vi "Main.vi"() -> ()   [LabVIEW 2017]
uses:
  1. CTL/State.ctl
  <vilib>/Utility/sysdir.llb/System Directory Type.ctl
  <vilib>/Instr/_visa.llb/VISA Configure Serial Port (Instr).vi
panel:
  in  "VISA resource name":refnum<visa-resource-name> caption="VISA 리소스 이름"
  out "String 3":string
  out "String 2":string
  out "String":string
  out "3회시험결과":string
  out "2회시험결과":string
  out "1회시험결과":string
  out "시험결과":string
  in  "데이터 저장":bool=TRUE
  in  "PNF ON":bool=TRUE
  in  "정지 버튼":bool=TRUE
  # "AUV Pinger TEST"
  # "시험 결과"
  # "COM 포트 설정"
  # "1회 시험 데이터"
  # "2회 시험 데이터"
  # "3회 시험 데이터"
  # "2회 시험 결과"
  # "3회 시험 결과"
  # "1회 시험 결과"
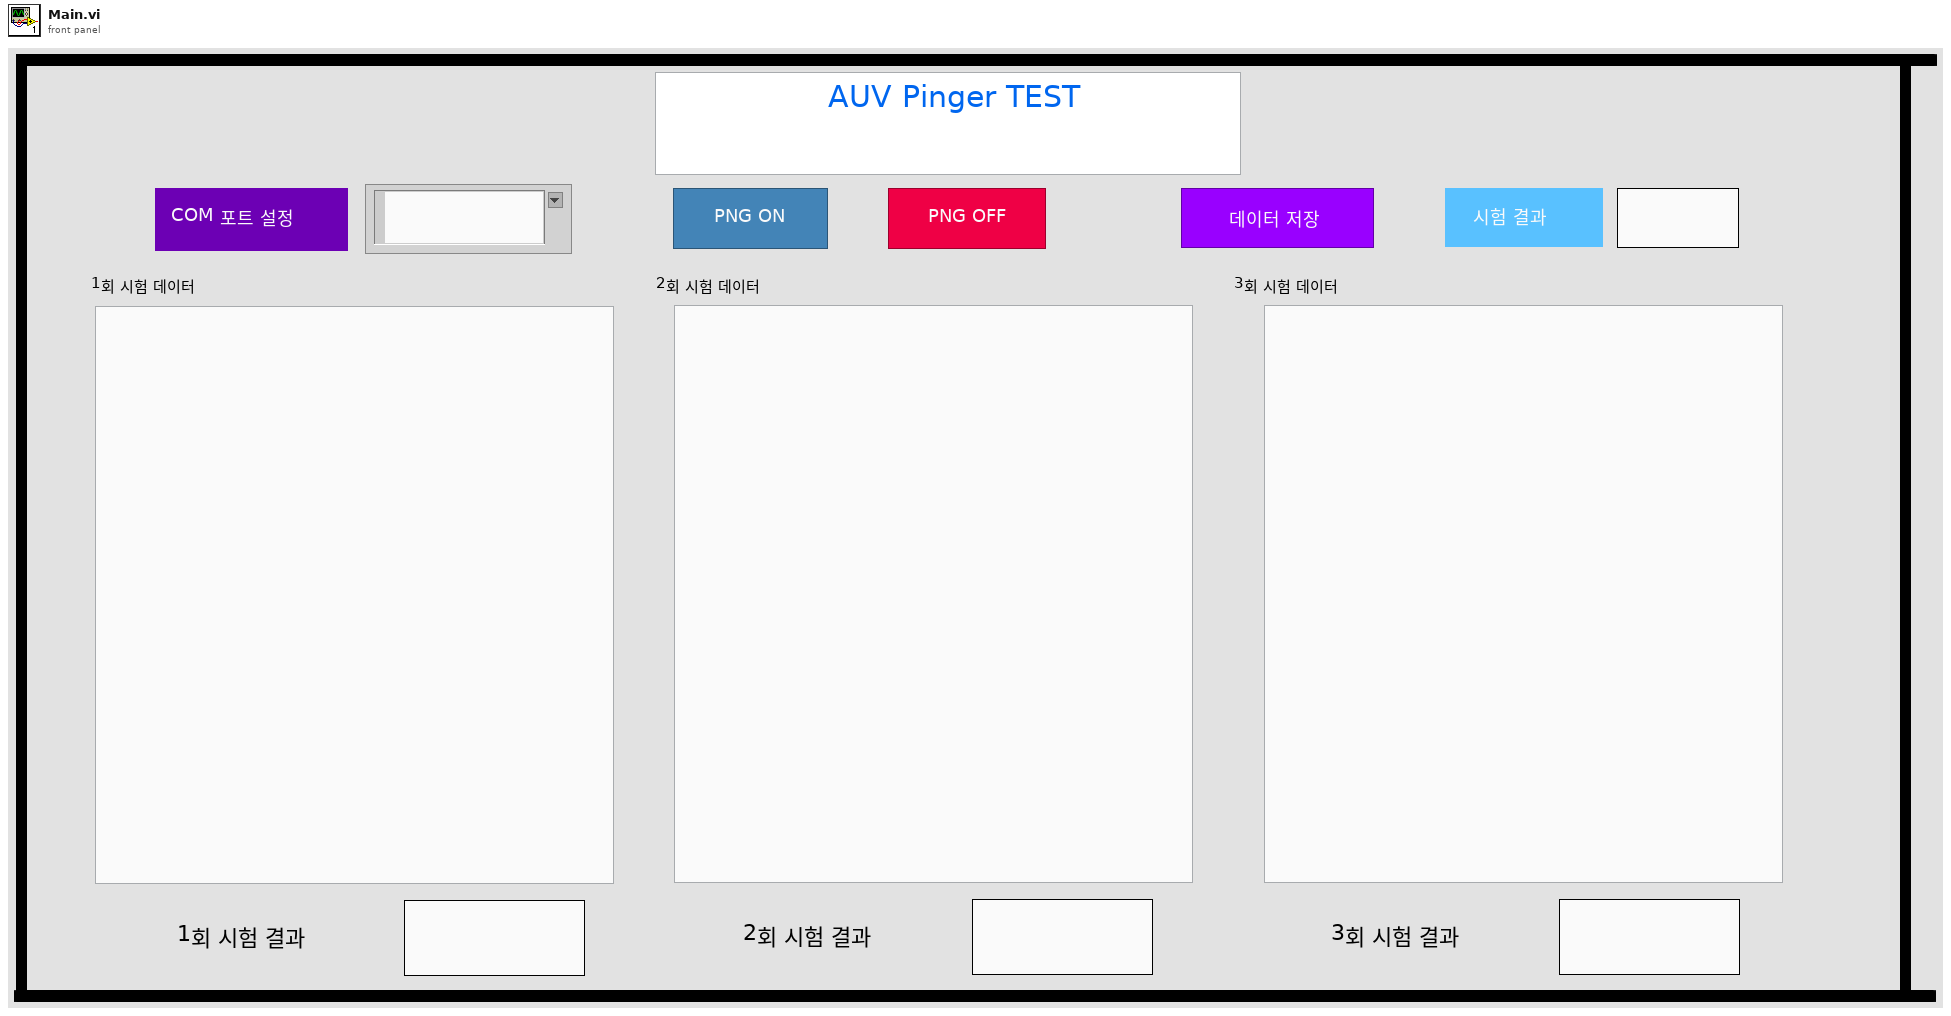
[diagram p1: front panel]
types:
  T1 = cluster{"1회 시험결과":string, "2회 시험결과":string, "3회 시험결과":string, "시험결과":string, "COM 포트":refnum<visa-resource-name>, "카운터":i32, "1회 로그":string, "2회 로그":string, "3회 로그":string, "1회 결과 카운트":i32, "2회 결과 카운트":i32, "3회 결과 카운트":i32}
  T2 = typedef "State.ctl" = enum16{"초기화", "시작", "정지", "데이터 저장"}
  T3 = enum16{"open", "replace", "create", "open or create", "replace or create", "replace or create with confirmation"}
  T4 = typedef "System Directory Type.ctl" = i32
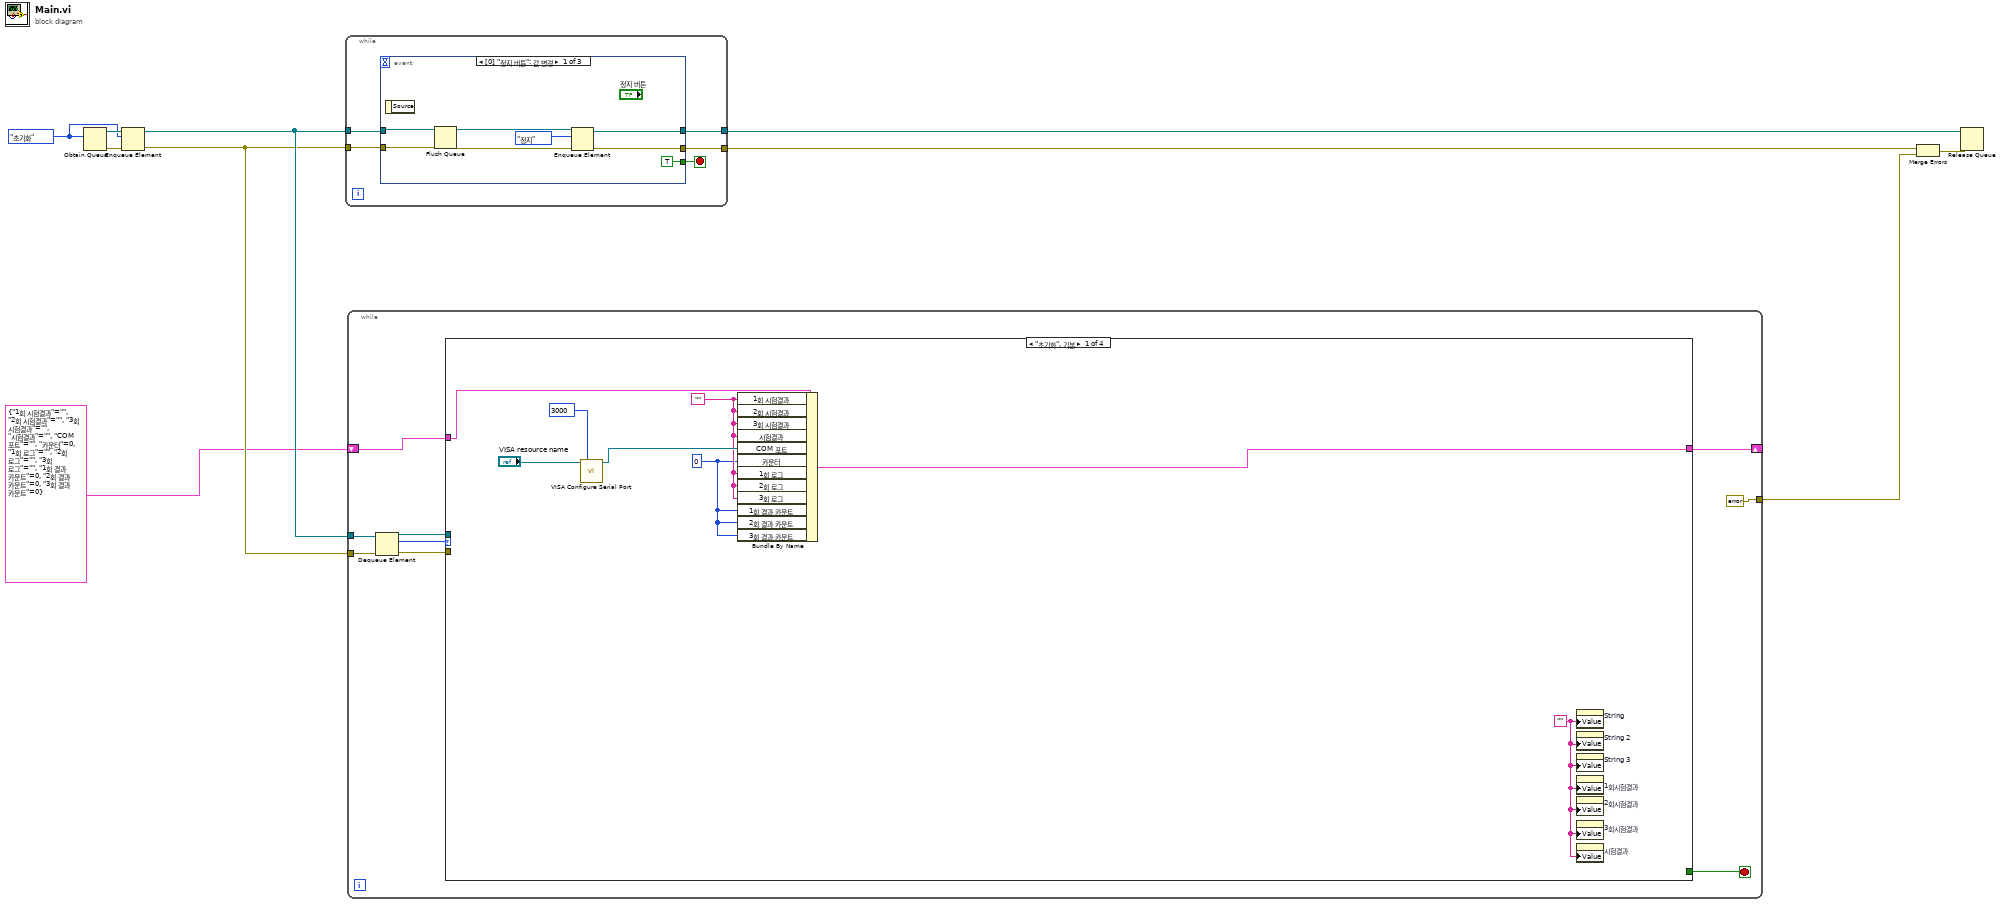
[diagram p0: block diagram]
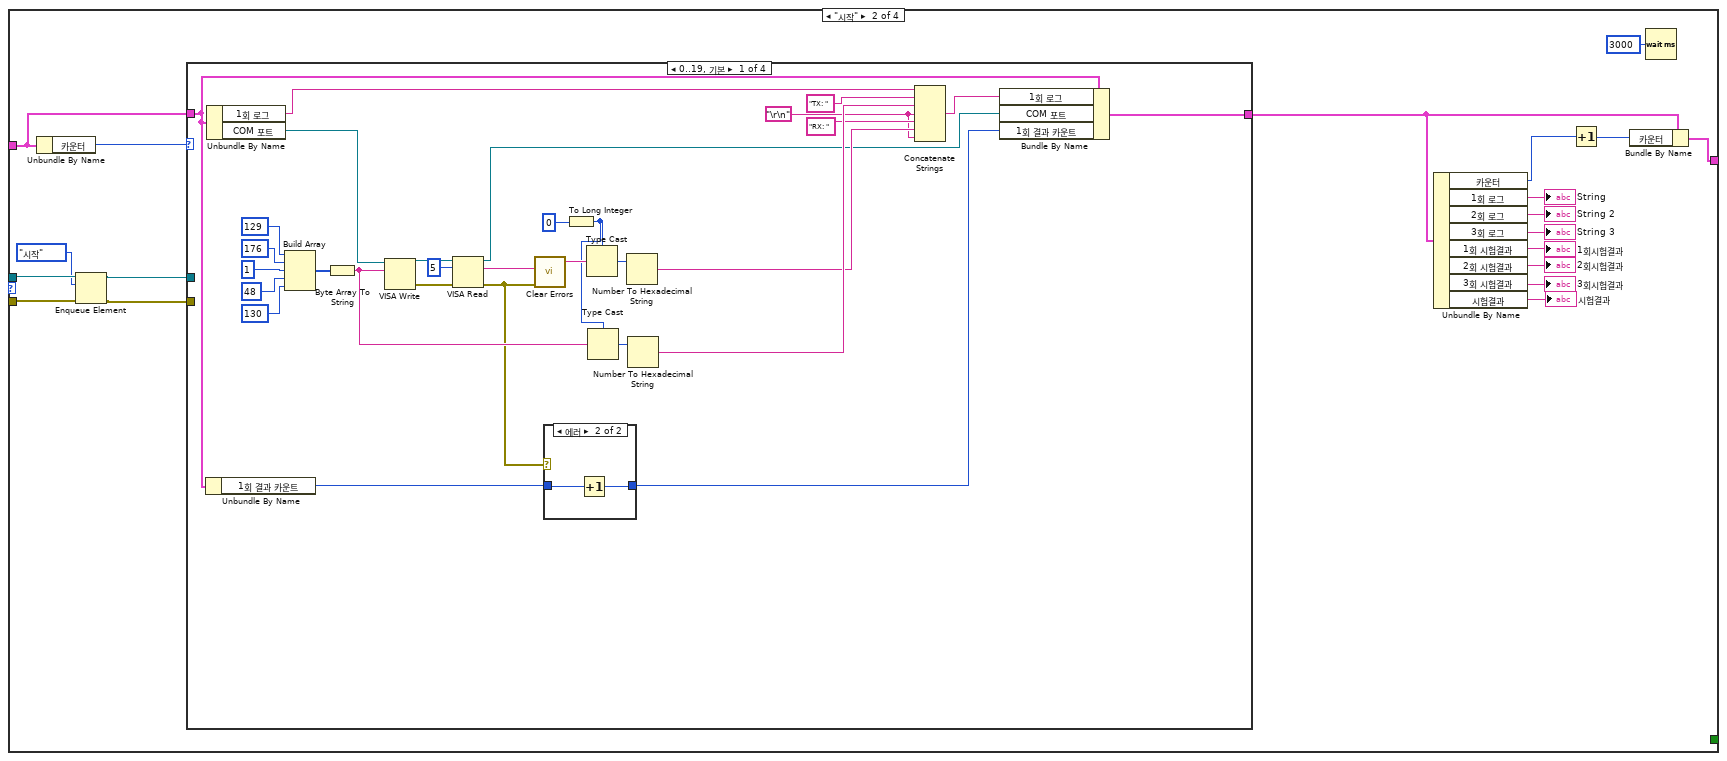
[diagram p2: hidden frame]
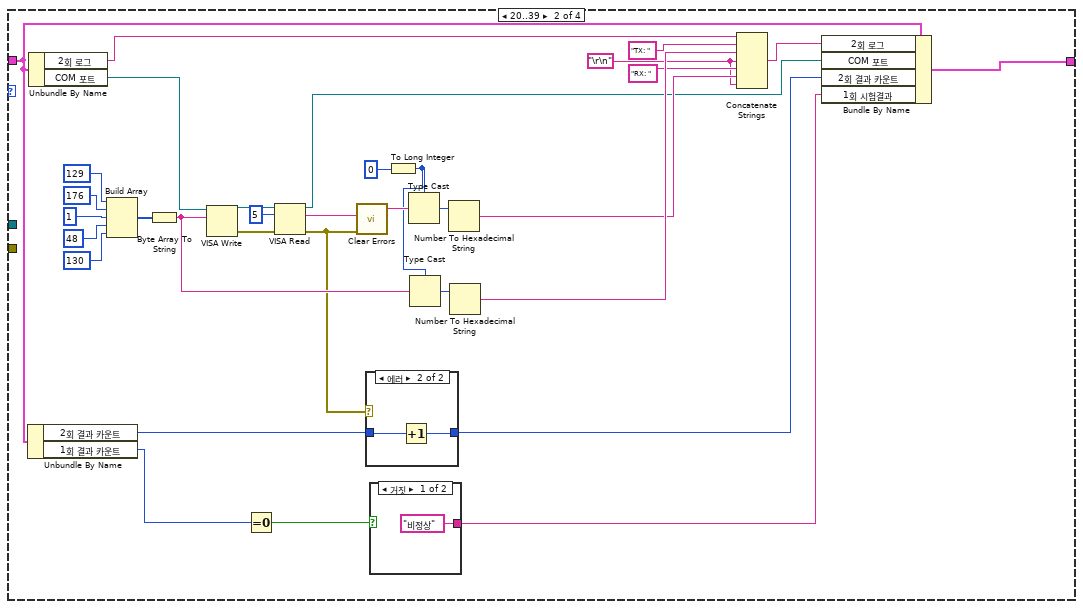
[diagram p4: hidden frame]
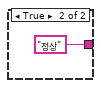
[diagram p5: hidden frame]
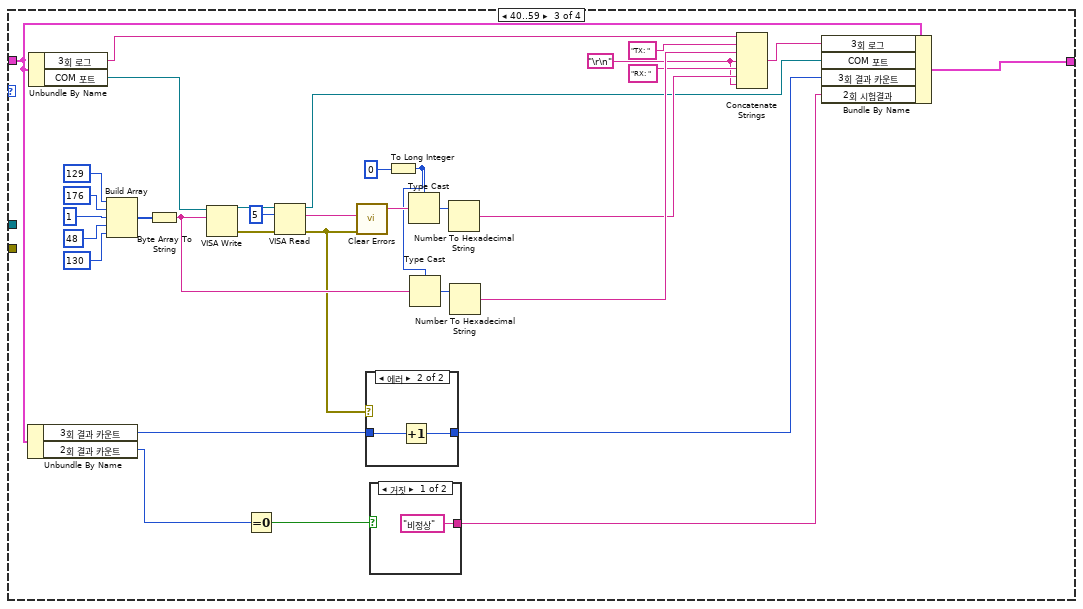
[diagram p7: hidden frame]
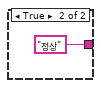
[diagram p8: hidden frame]
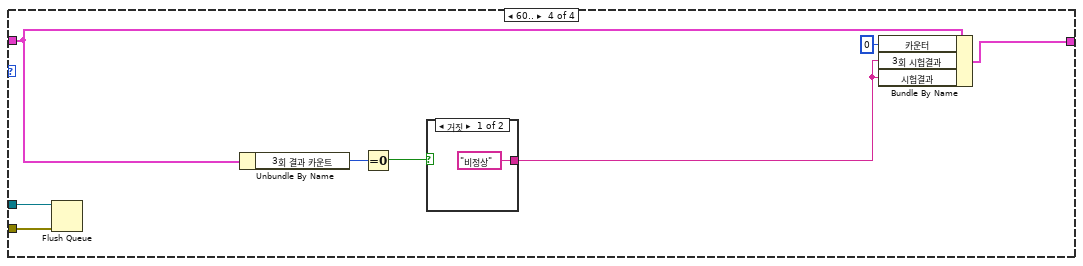
[diagram p10: hidden frame]
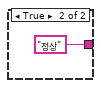
[diagram p11: hidden frame]
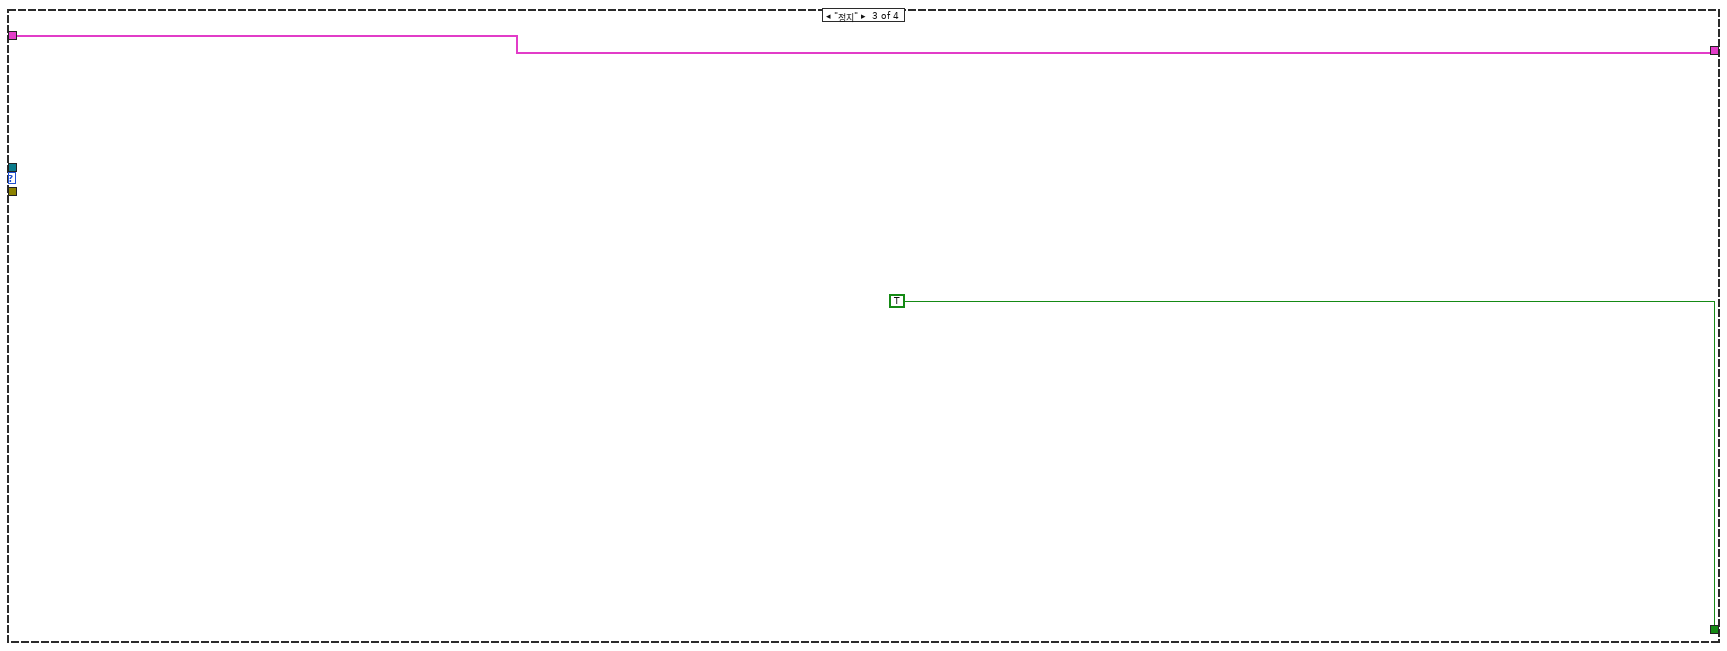
[diagram p12: hidden frame]
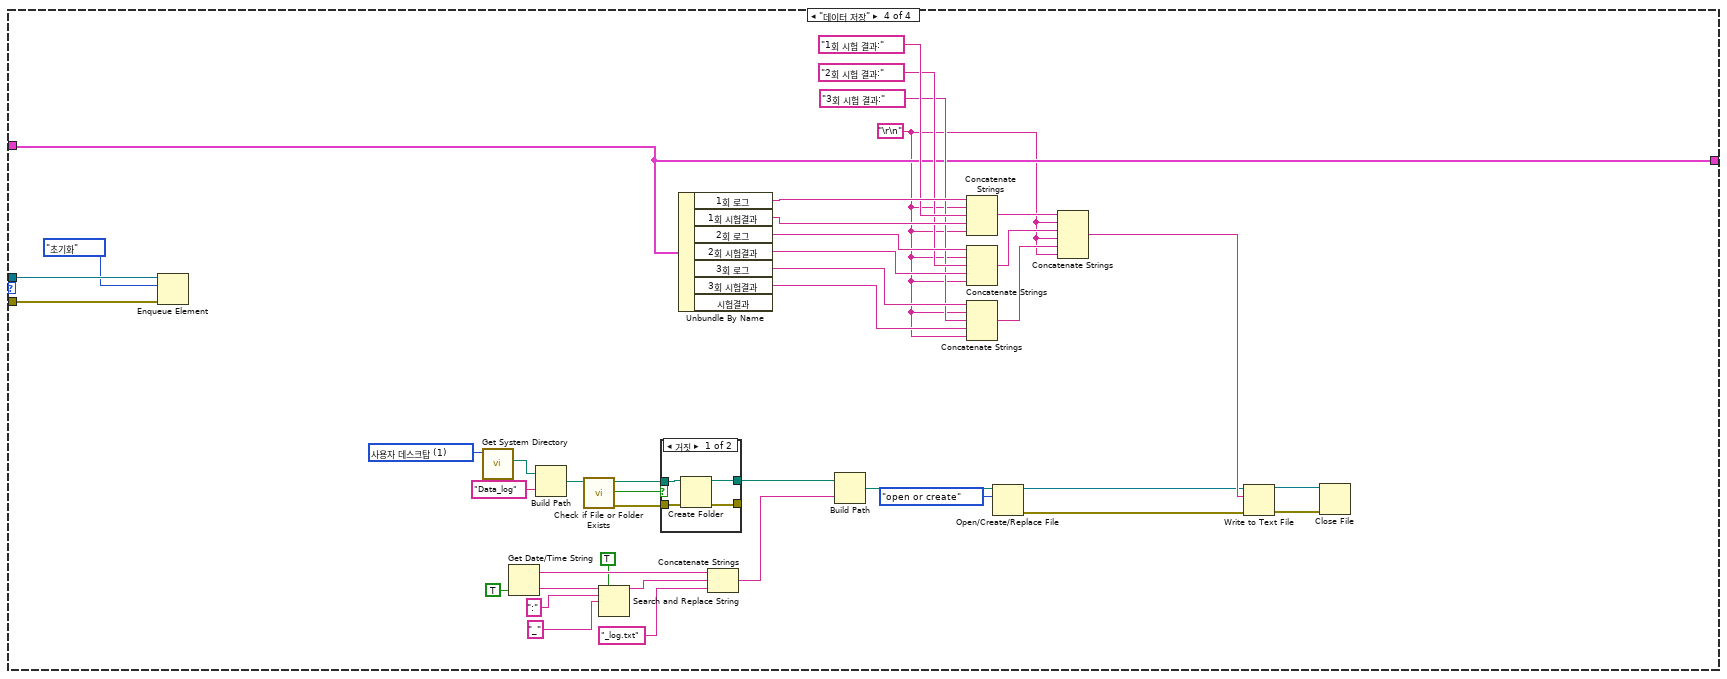
[diagram p13: hidden frame]
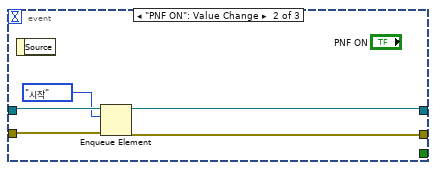
[diagram p15: hidden frame]
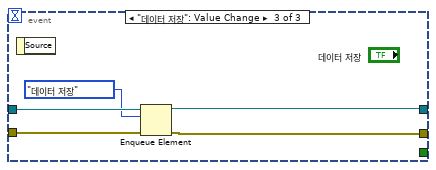
[diagram p16: hidden frame]
diagram:
  w8 = State."초기화"
  n1 = Obtain Queue(element data type=w8) -> (queue out=w10:refnum<queue>, error out=w9:errorcluster)  [unwired: 4 in, 1 out]
  n2 = Enqueue Element(queue=w10, element=w8, error in (no error)=w9) -> (queue out=w7:refnum<queue>, error out=w6:errorcluster)  [unwired: 1 in, 1 out]
  n3 = while {
    tunnel: w7 -> [w15]
    tunnel: w6 -> [w14]
    tunnel: [w12] -> w5
    tunnel: [w11] -> w2
    stop <- w13 stop-if-true
    n4 = event shown="[0] \"정지 버튼\": 값 변경" {
      selector: _ -> [_ _ _]
      dyn-events: _ -> [_ _ _]
      timeout: _ -> [_ _ _]
      tunnel: w15 -> [w16 w28 w33]
      tunnel: w14 -> [w17 w27 w32]
      tunnel: [TRUE _ _] -> w13
      tunnel: [w21 w24 w29] -> w12
      tunnel: [w20 w25 w30] -> w11
      event "정지 버튼": Value Change {
        n5 = event-data() -> ()  [unwired: 1 in, 1 out]
        n6 = Flush Queue(queue=w16, error in (no error)=w17) -> (queue out=w19:refnum<queue>, error out=w18:errorcluster)  [unwired: 1 out]
        n7 = Enqueue Element(queue=w19, element=State."정지", error in (no error)=w18) -> (queue out=w20:refnum<queue>, error out=w21:errorcluster)  [unwired: 1 in, 1 out]
      }
      event "PNF ON": Value Change {
        n8 = event-data() -> ()  [unwired: 1 in, 1 out]
        n9 = Enqueue Element(queue=w28, element=State."시작", error in (no error)=w27) -> (queue out=w25:refnum<queue>, error out=w24:errorcluster)  [unwired: 1 in, 1 out]
      }
      event "데이터 저장": Value Change {
        n10 = event-data() -> ()  [unwired: 1 in, 1 out]
        n11 = Enqueue Element(queue=w33, element=State."데이터 저장", error in (no error)=w32) -> (queue out=w30:refnum<queue>, error out=w29:errorcluster)  [unwired: 1 in, 1 out]
      }
    }
  }
  n12 = while {
    tunnel: w7 -> [w38]
    tunnel: w6 -> [w42]
    tunnel: [errorcluster {"status"=FALSE, "code"=0, "source"=""} ("에러 상수")] -> w4
    shift-right: [w34] -> _
    shift-left: T1 {"1회 시험결과"="", "2회 시험결과"="", "3회 시험결과"="", "시험결과"="", "COM 포트"="", "카운터"=0, "1회 로그"="", "2회 로그"="", "3회 로그"="", "1회 결과 카운트"=0, "2회 결과 카운트"=0, "3회 결과 카운트"=0} -> [w39]
    stop <- w41 stop-if-true
    n13 = Dequeue Element(queue=w38, error in (no error)=w42) -> (queue out=w36:refnum<queue>, element=w37:T2, error out=w35:errorcluster)  [unwired: 1 in, 1 out]
    n14 = case shown="\"초기화\", 기본" w37 {
      tunnel: [_ _ TRUE _] -> w41
      tunnel: w39 -> [w50 w68 w186 w204]
      tunnel: [w49 w61 w186 w204] -> w34
      tunnel: w36 -> [_ w60 _ w228]
      tunnel: w35 -> [_ w59 _ w227]
      frame "초기화", Default {
        w43 = 0
        w44 = ""
        w45 = ""
        n15 = call-poly "VISA Configure Serial Port"("VISA resource name"="VISA resource name", "timeout (10sec)"=u32 3000) -> ("VISA resource name out"=w47:refnum<visa-resource-name>)  [unwired: 12 in, 1 out]
        n16 = Bundle By Name(cluster=w50, "1회 시험결과"=w44, "2회 시험결과"=w44, "3회 시험결과"=w44, "시험결과"=w44, "COM 포트"=w47, "카운터"=w43, "1회 로그"=w44, "2회 로그"=w44, "3회 로그"=w44, "1회 결과 카운트"=w43, "2회 결과 카운트"=w43, "3회 결과 카운트"=w43) -> (w49:T1)
        n17 = property on="String" class="Str"("Value"=w45) -> ()  [unwired: 2 in, 2 out]
        n18 = property on="String 2" class="Str"("Value"=w45) -> ()  [unwired: 2 in, 2 out]
        n19 = property on="String 3" class="Str"("Value"=w45) -> ()  [unwired: 2 in, 2 out]
        n20 = property on="1회시험결과" class="Str"("Value"=w45) -> ()  [unwired: 2 in, 2 out]
        n21 = property on="2회시험결과" class="Str"("Value"=w45) -> ()  [unwired: 2 in, 2 out]
        n22 = property on="3회시험결과" class="Str"("Value"=w45) -> ()  [unwired: 2 in, 2 out]
        n23 = property on="시험결과" class="Str"("Value"=w45) -> ()  [unwired: 2 in, 2 out]
      }
      frame "시작" {
        n24 = Unbundle By Name(w68) -> ("카운터"=w69:i32)
        n25 = Enqueue Element(queue=w60, element=State."시작", error in (no error)=w59) -> (queue out=w57:refnum<queue>, error out=w56:errorcluster)  [unwired: 1 in, 1 out]
        n26 = case shown="0..19, 기본" w69 {
          tunnel: w68 -> [w72 w107 w144 w181]
          tunnel: [w97 w132 w169 w182] -> w66
          tunnel: w57 -> [_ _ _ w177]
          tunnel: w56 -> [_ _ _ w176]
          frame 0..19, Default {
            w77 = "\r\n"
            n27 = Unbundle By Name(w72) -> ("1회 결과 카운트"=w71:i32)
            n28 = Unbundle By Name(w72) -> ("1회 로그"=w84:string, "COM 포트"=w83:refnum<visa-resource-name>)
            n29 = Build Array(129, 176, 1, 48, 130) -> (w88:i32[])
            n30 = Byte Array To String(unsigned byte array=w88) -> (string=w82:string)
            n31 = VISA Write(VISA resource name=w83, write buffer=w82) -> (VISA resource name out=w96:refnum<visa-resource-name>, error out=w94:errorcluster)  [unwired: 1 in, 1 out]
            n32 = VISA Read(VISA resource name=w96, byte count=u32 5 ("바이트 카운트"), error in (no error)=w94) -> (VISA resource name out=w76:refnum<visa-resource-name>, read buffer=w87:string, error out=w73:errorcluster)  [unwired: 1 out]
            n33 = call <vilib>:"Clear Errors.vi"("error in (no error)"=w73) -> ()  [unwired: 5 in, 2 out]
            n34 = case shown="에러" w73 {
              tunnel: [w99 w101] -> w70
              tunnel: w71 -> [w99 w100]
              frame No Error {
              }
              frame Error {
                n35 = Increment(x=w100) -> (x+1=w101:i32)
              }
            }
            n36 = To Long Integer(number=0 ("숫자")) -> (32bit integer=w75:i32)
            n37 = Type Cast(type=w75, x=w87) -> (*(type *) &x=w86:i32)
            n38 = Type Cast(type=w75, x=w82) -> (*(type *) &x=w74:i32)
            n39 = Number To Hexadecimal String(2:w86) -> (0:w78:string)  [unwired: 1 in]
            n40 = Number To Hexadecimal String(2:w74) -> (0:w80:string)  [unwired: 1 in]
            n41 = Concatenate Strings(w84, "TX: ", w80, w77, "RX: ", w78, w77) -> (w98:string)
            n42 = Bundle By Name(cluster=w72, "1회 로그"=w98, "COM 포트"=w76, "1회 결과 카운트"=w70) -> (w97:T1)
          }
          frame 20..39 {
            w112 = "\r\n"
            n43 = Unbundle By Name(w107) -> ("2회 결과 카운트"=w106:i32, "1회 결과 카운트"=w104:i32)
            n44 = Unbundle By Name(w107) -> ("2회 로그"=w119:string, "COM 포트"=w118:refnum<visa-resource-name>)
            n45 = Build Array(129, 176, 1, 48, 130) -> (w123:i32[])
            n46 = Byte Array To String(unsigned byte array=w123) -> (string=w117:string)
            n47 = VISA Write(VISA resource name=w118, write buffer=w117) -> (VISA resource name out=w131:refnum<visa-resource-name>, error out=w129:errorcluster)  [unwired: 1 in, 1 out]
            n48 = Equal To 0?(x=w104) -> (x = 0?=w103:bool)
            n49 = VISA Read(VISA resource name=w131, byte count=u32 5 ("바이트 카운트"), error in (no error)=w129) -> (VISA resource name out=w111:refnum<visa-resource-name>, read buffer=w122:string, error out=w108:errorcluster)  [unwired: 1 out]
            n50 = call <vilib>:"Clear Errors.vi"("error in (no error)"=w108) -> ()  [unwired: 5 in, 2 out]
            n51 = case shown="에러" w108 {
              tunnel: [w136 w138] -> w105
              tunnel: w106 -> [w136 w137]
              frame No Error {
              }
              frame Error {
                n52 = Increment(x=w137) -> (x+1=w138:i32)
              }
            }
            n53 = case shown="거짓" w103 {
              tunnel: ["비정상" "정상"] -> w102
              frame False {
              }
              frame True {
              }
            }
            n54 = To Long Integer(number=0 ("숫자")) -> (32bit integer=w110:i32)
            n55 = Type Cast(type=w110, x=w122) -> (*(type *) &x=w121:i32)
            n56 = Type Cast(type=w110, x=w117) -> (*(type *) &x=w109:i32)
            n57 = Number To Hexadecimal String(2:w121) -> (0:w113:string)  [unwired: 1 in]
            n58 = Number To Hexadecimal String(2:w109) -> (0:w115:string)  [unwired: 1 in]
            n59 = Concatenate Strings(w119, "TX: ", w115, w112, "RX: ", w113, w112) -> (w133:string)
            n60 = Bundle By Name(cluster=w107, "2회 로그"=w133, "COM 포트"=w111, "2회 결과 카운트"=w105, "1회 시험결과"=w102) -> (w132:T1)
          }
          frame 40..59 {
            w149 = "\r\n"
            n61 = Unbundle By Name(w144) -> ("3회 결과 카운트"=w143:i32, "2회 결과 카운트"=w141:i32)
            n62 = Unbundle By Name(w144) -> ("3회 로그"=w156:string, "COM 포트"=w155:refnum<visa-resource-name>)
            n63 = Build Array(129, 176, 1, 48, 130) -> (w160:i32[])
            n64 = Byte Array To String(unsigned byte array=w160) -> (string=w154:string)
            n65 = VISA Write(VISA resource name=w155, write buffer=w154) -> (VISA resource name out=w168:refnum<visa-resource-name>, error out=w166:errorcluster)  [unwired: 1 in, 1 out]
            n66 = Equal To 0?(x=w141) -> (x = 0?=w140:bool)
            n67 = VISA Read(VISA resource name=w168, byte count=u32 5 ("바이트 카운트"), error in (no error)=w166) -> (VISA resource name out=w148:refnum<visa-resource-name>, read buffer=w159:string, error out=w145:errorcluster)  [unwired: 1 out]
            n68 = call <vilib>:"Clear Errors.vi"("error in (no error)"=w145) -> ()  [unwired: 5 in, 2 out]
            n69 = case shown="에러" w145 {
              tunnel: [w173 w175] -> w142
              tunnel: w143 -> [w173 w174]
              frame No Error {
              }
              frame Error {
                n70 = Increment(x=w174) -> (x+1=w175:i32)
              }
            }
            n71 = case shown="거짓" w140 {
              tunnel: ["비정상" "정상"] -> w139
              frame False {
              }
              frame True {
              }
            }
            n72 = To Long Integer(number=0 ("숫자")) -> (32bit integer=w147:i32)
            n73 = Type Cast(type=w147, x=w159) -> (*(type *) &x=w158:i32)
            n74 = Type Cast(type=w147, x=w154) -> (*(type *) &x=w146:i32)
            n75 = Number To Hexadecimal String(2:w158) -> (0:w150:string)  [unwired: 1 in]
            n76 = Number To Hexadecimal String(2:w146) -> (0:w152:string)  [unwired: 1 in]
            n77 = Concatenate Strings(w156, "TX: ", w152, w149, "RX: ", w150, w149) -> (w170:string)
            n78 = Bundle By Name(cluster=w144, "3회 로그"=w170, "COM 포트"=w148, "3회 결과 카운트"=w142, "2회 시험결과"=w139) -> (w169:T1)
          }
          frame 60.. {
            n79 = Flush Queue(queue=w177, error in (no error)=w176) -> ()  [unwired: 3 out]
            n80 = Unbundle By Name(w181) -> ("3회 결과 카운트"=w180:i32)
            n81 = Equal To 0?(x=w180) -> (x = 0?=w179:bool)
            n82 = case shown="거짓" w179 {
              tunnel: ["비정상" "정상"] -> w178
              frame False {
              }
              frame True {
              }
            }
            n83 = Bundle By Name(cluster=w181, "카운터"=0, "3회 시험결과"=w178, "시험결과"=w178) -> (w182:T1)
          }
        }
        n84 = Unbundle By Name(w66) -> ("카운터"=w67:i32, "1회 로그"=→"String":string, "2회 로그"=→"String 2":string, "3회 로그"=→"String 3":string, "1회 시험결과"=→"1회시험결과":string, "2회 시험결과"=→"2회시험결과":string, "3회 시험결과"=→"3회시험결과":string, "시험결과"=→"시험결과":string)
        n85 = Increment(x=w67) -> (x+1=w65:i32)
        n86 = Bundle By Name(cluster=w66, "카운터"=w65) -> (w61:T1)
        n87 = Wait (ms)(milliseconds to wait=u32 3000 ("대기 시간 (ms)")) -> ()  [unwired: 1 out]
      }
      frame "정지" {
      }
      frame "데이터 저장" {
        w188 = "\r\n"
        w225 = T4 1 items=["사용자 홈"=0, "사용자 데스크탑"=1, "사용자 문서"=2, "사용자 어플리케이션 데이터"=3, "사용자 환경"=4, "사용자 임시"=5, "퍼블릭 문서"=6, "퍼블릭 어플리케이션 데이터"=7, "퍼블릭 환경"=8, "퍼블릭 캐시"=13, "시스템 코어 라이브러리"=9, "시스템 설치된 라이브러리"=10, "어플리케이션 파일"=11, "부팅 볼륨 루트"=12] ("system directory type")
        n88 = Enqueue Element(queue=w228, element=State."초기화", error in (no error)=w227) -> ()  [unwired: 1 in, 3 out]
        n89 = call <vilib>:"Get System Directory.vi"("system directory type"=w225) -> ("system directory"=w224:path)  [unwired: 10 in]
        n90 = Get Date/Time String(want seconds? (F)=TRUE ("초 보이기? (거짓)")) -> (date string=w193:string, time string=w197:string)  [unwired: 2 in]
        n91 = Build Path(base path=w224, name or relative path="Data_log" ("이름 또는 상대 경로")) -> (appended path=w222:path)
        n92 = call <vilib>:"Check if File or Folder Exists.vi"("path"=w222) -> ("error out"=w219:errorcluster, "file or folder exists?"=w221:bool, "dup path"=w220:path)  [unwired: 8 in]
        n93 = Search and Replace String(replace all?=TRUE ("모두 대체? (거짓)"), input string=w197, search string=":" ("검색 문자열"), replace string="_" ("대체 문자열(\"\")")) -> (result string=w194:string)  [unwired: 4 in, 3 out]
        n94 = case shown="거짓" w221 {
          tunnel: w220 -> [w232 w234]
          tunnel: w219 -> [w231 w233]
          tunnel: [w230 w234] -> w218
          tunnel: [w229 w233] -> _
          frame False {
            n95 = Create Folder(path (use dialog)=w232, error in=w231) -> (created path=w230:path, error out=w229:errorcluster)  [unwired: 1 in, 1 out]
          }
          frame True {
          }
        }
        n96 = Unbundle By Name(w204) -> ("1회 로그"=w217:string, "1회 시험결과"=w215:string, "2회 로그"=w214:string, "2회 시험결과"=w212:string, "3회 로그"=w211:string, "3회 시험결과"=w209:string)  [unwired: 1 out]
        n97 = Concatenate Strings(w193, w194, "_log.txt") -> (w191:string)
        n98 = Build Path(base path=w218, name or relative path=w191) -> (appended path=w203:path)
        n99 = Concatenate Strings(w217, w188, "1회 시험 결과:", w215, w188) -> (w208:string)
        n100 = Concatenate Strings(w214, w188, "2회 시험 결과:", w212, w188) -> (w190:string)
        n101 = Concatenate Strings(w211, w188, "3회 시험 결과:", w209, w188) -> (w189:string)
        n102 = Open/Create/Replace File(file path (use dialog)=w203, operation (0:open)=T3."open or create" ("동작(0:open)")) -> (refnum out=w202:refnum<file>, error out=w201:errorcluster)  [unwired: 4 in, 1 out]
        n103 = Concatenate Strings(w208, w188, w190, w188, w189, w188) -> (w207:string)
        n104 = Write to Text File(file (use dialog)=w202, text=w207, error in=w201) -> (refnum out=w206:refnum<file>, error out=w205:errorcluster)  [unwired: 1 in, 1 out]
        n105 = Close File(refnum=w206, error in=w205) -> ()  [unwired: 2 out]
      }
    }
  }
  n106 = Merge Errors(w5, w4) -> (w3:errorcluster)
  n107 = Release Queue(queue=w2, error in (no error)=w3) -> ()  [unwired: 1 in, 3 out]
